vi "isEnabled.vi"(8 "error in (no error)":errorcluster, 11 "Radio in":refnum<class "Radio.lvclass">) -> (0 "error out":errorcluster, 2 "on":bool, 3 "Radio out":refnum<class "Radio.lvclass">)   [LabVIEW 2018, in "Radio.lvclass"]
uses:
  Radio.lvclass
  Radio.lvclass/Radio.ctl
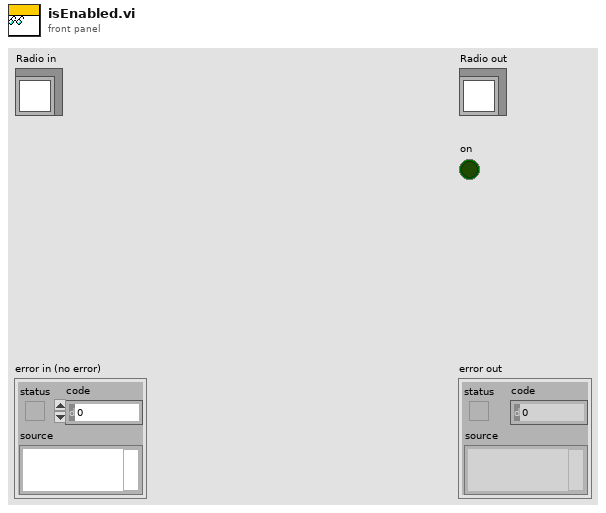
[diagram p1: front panel]
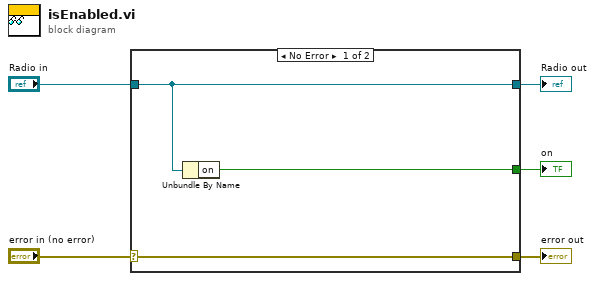
[diagram p0: block diagram]
diagram:
  n1 = case shown="No Error" "error in (no error)" {
    selector: "error in (no error)" -> [w8 w9]
    tunnel: [w8 w9] -> w4
    tunnel: [w7 w10] -> w2
    tunnel: "Radio in" -> [w7 w10]
    tunnel: [w6 _] -> w1
    frame No Error {
      n2 = Unbundle By Name(w7) -> ("on"=w6:bool)
    }
    frame Error {
    }
  }
  "error out" <- w4
  "Radio out" <- w2
  "on" <- w1
